vi "outref.vi"(1 "error in (no error)":errorcluster) -> (14 "VI out":refnum<vi>, 15 "error out":errorcluster)   [LabVIEW 2015]
panel:
  in  "stop":bool
  out "appended path":path
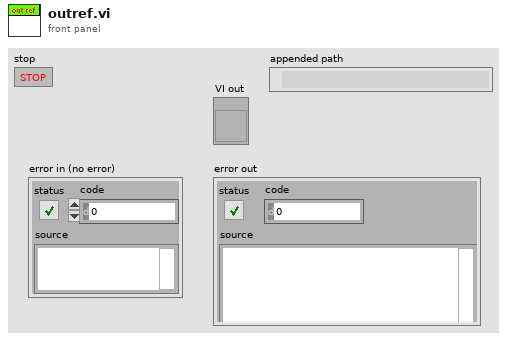
[diagram p1: front panel]
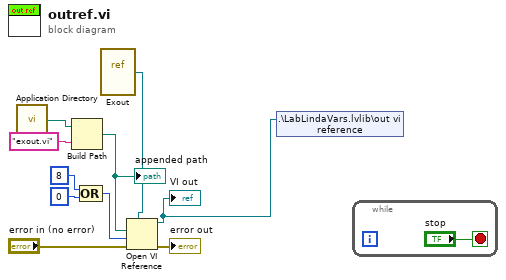
[diagram p0: block diagram]
diagram:
  n1 = call <vilib>:"Application Directory.vi"() -> ("Application Directory"=w3:path)
  n2 = Build Path(base path=w3, name or relative path="exout.vi") -> (appended path=w5:path)
  "appended path" <- w5
  n3 = Compound Arithmetic op=OR(8 ("options"), 0 ("value")) -> (w8:i32)
  n4 = vi-ref "Exout.vi"() -> (w2:refnum<vi>)
  n5 = Open VI Reference(type specifier VI Refnum (for type only)=w2, vi path=w5, options=w8, error in (no error)="error in (no error)") -> (vi reference=w1:refnum<vi>, error out=→"error out":errorcluster)  [unwired: 2 in]
  "VI out" <- w1
  n6 = shared-variable ".\\LabLindaVars.lvlib\\out vi reference"(w1) -> ()  [unwired: 1 in, 1 out]
  n7 = while {
    stop <- "stop" stop-if-true
  }
